vi "Encrypt Letter (Var-wrong).vi"(8 "error in":errorcluster, 10 "letter":string, 11 "Variant in":variant) -> (0 "error out":errorcluster, 2 "encrypted letter":string, 3 "Variant out":variant)   [LabVIEW 2015]
uses:
  Letter/Letter.lvclass
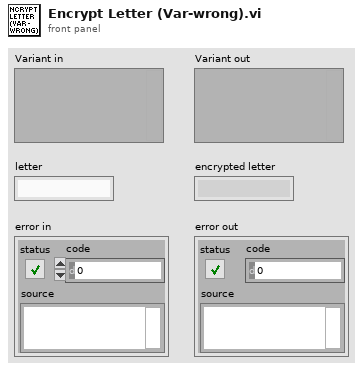
[diagram p1: front panel]
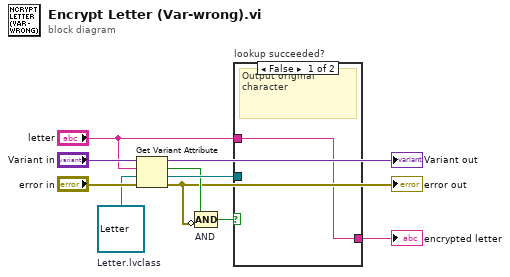
[diagram p0: block diagram]
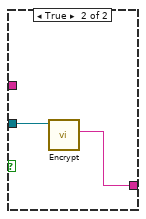
[diagram p2: hidden frame]
diagram:
  w2 = refnum<class "Letter.lvclass"> refnum  # Letter.lvclass
  n1 = Get Variant Attribute(Variant="Variant in", name="letter", default value (empty Variant)=w2, error in="error in") -> (duplicate Variant=→"Variant out":variant, found=w7:bool, value=w8:refnum<class "Letter.lvclass">, error out=w1:errorcluster)
  "error out" <- w1
  n2 = Compound Arithmetic op=AND "AND"(w7, invert w1) -> (w6:bool)
  n3 = case "lookup succeeded?" shown="False" w6 {
    tunnel: w8 -> [_ w12]
    tunnel: [w11 w13] -> w4
    tunnel: "letter" -> [w11 _]
    frame False {
      # "Output original character"
    }
    frame True {
      n4 = call "Encrypt.vi"("Letter in"=w12) -> ("letter"=w13:string)  [unwired: 9 in, 1 out]
    }
  }
  "encrypted letter" <- w4
